vi "external cmd - list files.vi"() -> (4 "files array":path[](array[path]))   [LabVIEW 2010]
uses:
  <vilib>/Utility/sysdir.llb/System Directory Type.ctl
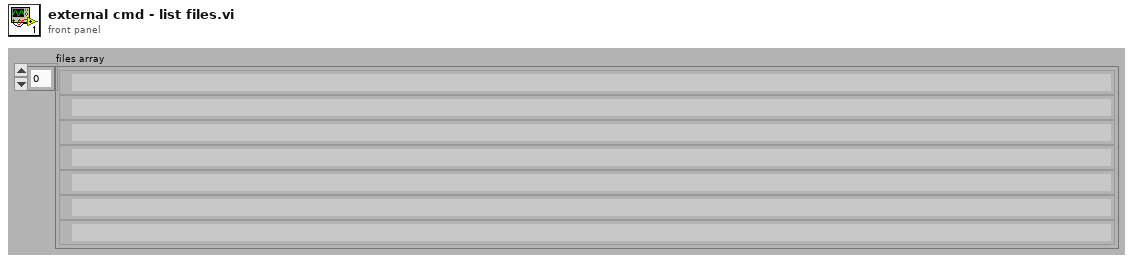
[diagram p1: front panel]
types:
  T1 = typedef "System Directory Type.ctl" = i32
  T2 = cluster{"last mod":timestamp, "appended path":path}
  T3 = cluster{"last mod":timestamp, "appended path":path}[]
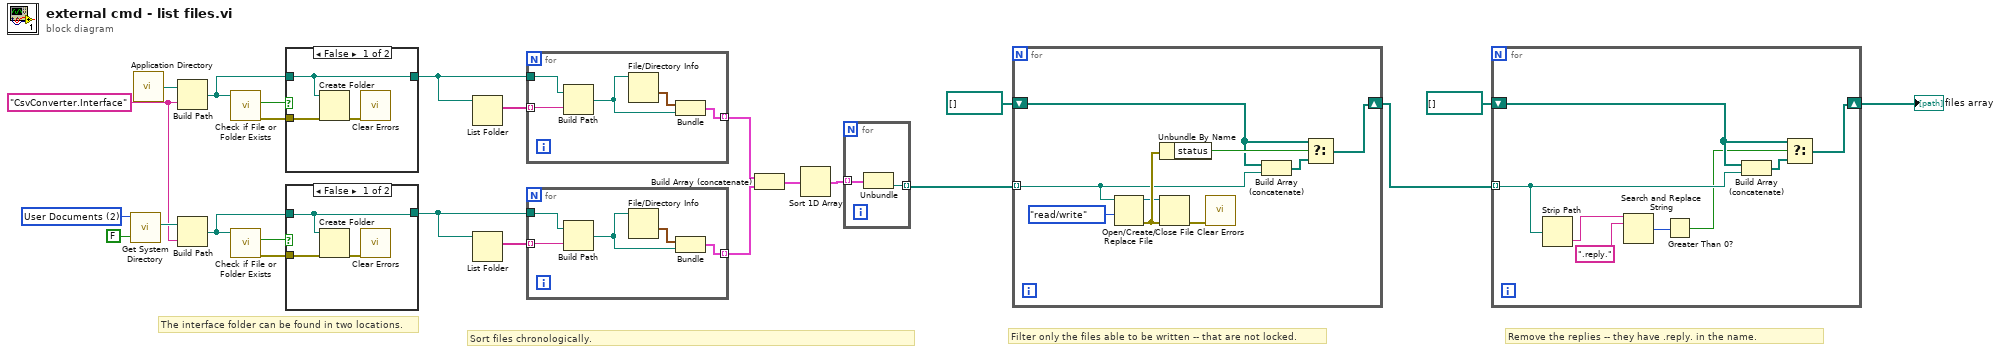
[diagram p0: block diagram]
diagram:
  w19 = T1 2 items=["User Home"=0, "User Desktop"=1, "User Documents"=2, "User Application Data"=3, "User Preferences"=4, "User Temporary"=5, "Public Documents"=6, "Public Application Data"=7, "Public Preferences"=8, "Public Cache"=13, "System Core Libraries"=9, "System Installed Libraries"=10, "Application Files"=11, "Boot Volume Root"=12] ("system directory type")
  w18 = "CsvConverter.Interface" ("name or relative path")
  # "Remove the replies -- they have .reply. in the name."
  # "Filter only the files able to be written -- that are not locked."
  # "Sort files chronologically."
  # "The interface folder can be found in two locations."
  n1 = call <vilib>:"Get System Directory.vi"("create directory if not found? (F)"=FALSE, "system directory type"=w19) -> ("system directory"=w21:path)  [unwired: 9 in]
  n2 = call <vilib>:"Application Directory.vi"() -> ("Application Directory"=w24:path)
  n3 = Build Path(base path=w24, name or relative path=w18) -> (appended path=w14:path)
  n4 = Build Path(base path=w21, name or relative path=w18) -> (appended path=w15:path)
  n5 = call <vilib>:"Check if File or Folder Exists.vi"("path"=w14) -> ("error out"=w23:errorcluster, "file or folder exists?"=w22:bool)  [unwired: 8 in, 1 out]
  n6 = call <vilib>:"Check if File or Folder Exists.vi"("path"=w15) -> ("error out"=w16:errorcluster, "file or folder exists?"=w17:bool)  [unwired: 8 in, 1 out]
  n7 = case shown="False" w22 {
    tunnel: w23 -> [w26 _]
    tunnel: w14 -> [w25 w28]
    tunnel: [w25 w28] -> w5
    frame False {
      n8 = Create Folder(path (use dialog)=w25, error in=w26) -> (error out=w27:errorcluster)  [unwired: 1 in, 2 out]
      n9 = call <vilib>:"Clear Errors.vi"("error in (no error)"=w27) -> ()  [unwired: 6 in, 1 out]
    }
    frame True {
    }
  }
  n10 = case shown="False" w17 {
    tunnel: w16 -> [w30 _]
    tunnel: w15 -> [w29 w32]
    tunnel: [w29 w32] -> w8
    frame False {
      n11 = Create Folder(path (use dialog)=w29, error in=w30) -> (error out=w31:errorcluster)  [unwired: 1 in, 2 out]
      n12 = call <vilib>:"Clear Errors.vi"("error in (no error)"=w31) -> ()  [unwired: 6 in, 1 out]
    }
    frame True {
    }
  }
  n13 = List Folder(path=w5) -> (filenames=w6:string[])  [unwired: 3 in, 3 out]
  n14 = List Folder(path=w8) -> (filenames=w7:string[])  [unwired: 3 in, 3 out]
  n15 = for {
    tunnel: w5 -> [w34]
    tunnel: [w36] -> w4 mode=indexing
    tunnel: w6 -> [w35] mode=indexing
    n16 = Build Path(base path=w34, name or relative path=w35) -> (appended path=w33:path)
    n17 = File/Directory Info(path=w33) -> (last mod=w37:timestamp)  [unwired: 1 in, 6 out]
    n18 = Bundle("last mod"=w37, "appended path"=w33) -> (w36:T2)  [unwired: 1 in]
  }
  n19 = for {
    tunnel: w8 -> [w39]
    tunnel: [w41] -> w12 mode=indexing
    tunnel: w7 -> [w40] mode=indexing
    n20 = Build Path(base path=w39, name or relative path=w40) -> (appended path=w38:path)
    n21 = File/Directory Info(path=w38) -> (last mod=w42:timestamp)  [unwired: 1 in, 6 out]
    n22 = Bundle("last mod"=w42, "appended path"=w38) -> (w41:T2)  [unwired: 1 in]
  }
  n23 = Build Array (concatenate)(w4, w12) -> (w11:T3)
  n24 = Sort 1D Array(array=w11) -> (sorted array=w13:T3)
  n25 = for {
    tunnel: w13 -> [w44] mode=indexing
    tunnel: [w43] -> w10 mode=indexing
    n26 = Unbundle(w44) -> ("appended path"=w43:path)  [unwired: 1 out]
  }
  n27 = for {
    tunnel: w10 -> [w47] mode=indexing
    shift-right: [w49] -> w2
    shift-left: path[] [] -> [w48]
    n28 = Open/Create/Replace File(file path (use dialog)=w47, access (0:read/write)=enum16{"read/write", "read-only", "write-only"}."read/write") -> (refnum out=w45:refnum<file>, error out=w52:errorcluster)  [unwired: 4 in, 1 out]
    n29 = Unbundle By Name(w52) -> ("status"=w50:bool)
    n30 = Close File(refnum=w45, error in=w52) -> (error out=w51:errorcluster)  [unwired: 1 out]
    n31 = call <vilib>:"Clear Errors.vi"("error in (no error)"=w51) -> ()  [unwired: 6 in, 1 out]
    n32 = Build Array (concatenate)(w48, w47) -> (w46:path[])
    n33 = Select(t=w48, s=w50, f=w46) -> (s? t:f=w49:path[])
  }
  n34 = for {
    tunnel: w2 -> [w58] mode=indexing
    shift-right: [w61] -> w1
    shift-left: path[] [] -> [w60]
    n35 = Strip Path(path=w58) -> (name=w57:string)  [unwired: 1 out]
    n36 = Search and Replace String(input string=w57, search string=".reply.") -> (number of replacements=w55:i32)  [unwired: 6 in, 3 out]
    n37 = Greater Than 0?(x=w55) -> (x > 0?=w54:bool)
    n38 = Build Array (concatenate)(w60, w58) -> (w59:path[])
    n39 = Select(t=w60, s=w54, f=w59) -> (s? t:f=w61:path[])
  }
  "files array" <- w1
